vi "SMTP Email MIME Send Header.vi"(4 "error in (no error)":errorcluster, 5 "MIME content-transfer-encoding (7bit)":string="7bit", 6 "MIME content-type (multipart/mixed)":string="multipart/mixed; boundary=\"LabVIEW_SMTP_MIME_Boundary\"", 7 "smtp session":T1) -> (0 "error out":errorcluster, 3 "smtp session out":T1)   [LabVIEW 2011, in "NewNI_SMTPEmail.lvlib"]
uses:
  NewNI_SMTPEmail.lvlib
  SMTP Email Session.ctl
panel:
  in  "buffered tcp connection":refnum<k5>
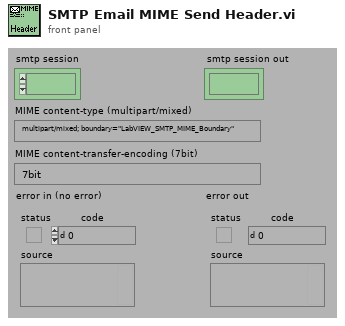
[diagram p1: front panel]
types:
  T1 = typedef "NewNI_SMTPEmail.lvlib/SMTP Email Session.ctl" = refnum<k1>
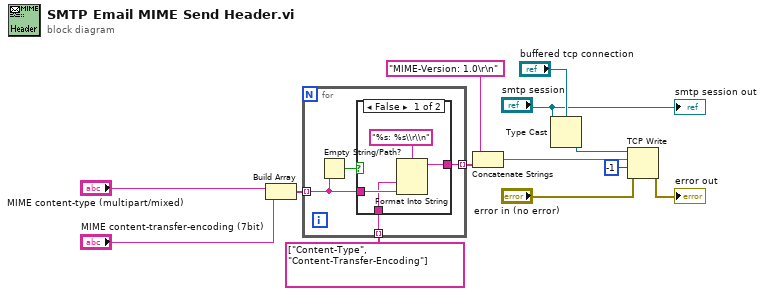
[diagram p0: block diagram]
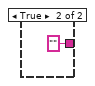
[diagram p2: hidden frame]
diagram:
  n1 = Build Array("MIME content-type (multipart/mixed)", "MIME content-transfer-encoding (7bit)") -> (w9:string[])
  n2 = for {
    tunnel: w9 -> [w16] mode=indexing
    tunnel: string[] ["Content-Type", "Content-Transfer-Encoding"] -> [w15] mode=indexing
    tunnel: [w14] -> w7 mode=indexing
    n3 = Empty String/Path?(string/path=w16) -> (empty?=w17:bool)
    n4 = case shown="False" w17 {
      tunnel: w16 -> [w20 _]
      tunnel: w15 -> [w19 _]
      tunnel: [w18 ""] -> w14
      frame False {
        n5 = Format Into String(format string="%s: %s\\r\\n", w19, w20) -> (resulting string=w18:string)  [unwired: 2 in, 1 out]
      }
      frame True {
      }
    }
  }
  n6 = Concatenate Strings("MIME-Version: 1.0\r\n", w7) -> (w5:string)
  n7 = Type Cast(type="buffered tcp connection", x="smtp session") -> (*(type *) &x=w2:refnum<k5>)
  n8 = TCP Write(connection ID=w2, data in=w5, error in (no error)="error in (no error)", 9:-1 ("timeout ms (25000)")) -> (error out=→"error out":errorcluster)  [unwired: 2 out]
  "smtp session out" <- "smtp session"
